vi "INTEGRATION TEST - Legacy Support.vi"(8 "error in (no error)":errorcluster) -> (0 "error out":errorcluster, 2 "Passed":bool)   [LabVIEW 2020, in "test_openg_variant_config_file.lvlib"]
uses:
  test_openg_variant_config_file.lvlib
  <vilib>/Utility/config.llb/NI_LVConfig.lvlib
  source/library/openg_variant_configuration_file.lvlib
  <userlib>/_OpenG.lib/file/file.llb/openg_file.lvlib
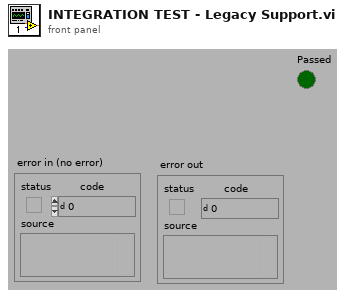
[diagram p1: front panel]
types:
  T1 = typedef "NI_LVConfig.lvlib/Config Data RefNum.ctl" = refnum<k1>
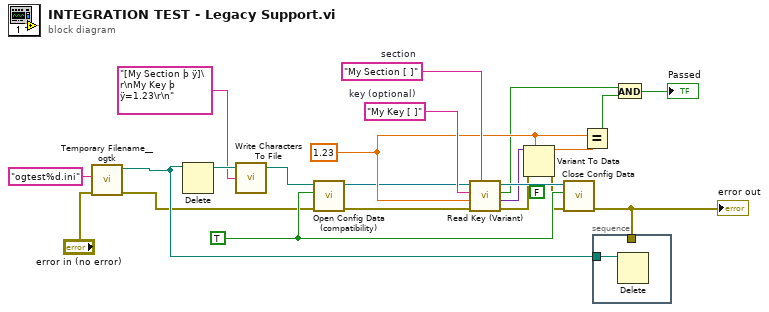
[diagram p0: block diagram]
diagram:
  (unwired) FALSE ("write configuration file? (T)")
  w15 = 1.23 ("Numeric")
  w21 = "My Key [ ]"  # key (optional)
  w22 = "My Section [ ]"  # section
  w19 = TRUE ("create file if necessary? (T)")
  n1 = call <userlib>:"Temporary Filename__ogtk.vi"("error in (no error)"="error in (no error)", "pattern (lvtemp%d.tmp)"="ogtest%d.ini") -> ("error out"=w2:errorcluster, "file in tmp dir"=w3:path)  [unwired: 4 in]
  n2 = Delete(path (use dialog)=w3) -> (deleted path=w9:path)  [unwired: 4 in, 2 out]
  n3 = call <vilib>:"Write Characters To File.vi"("character string"="[My Section þ ÿ]\r\nMy Key þ ÿ=1.23\r\n", "file path (dialog if empty)"=w9) -> ("new file path (Not A Path if cancelled)"=w8:path)  [unwired: 3 in]
  n4 = call <vilib>:"Open Config Data (compatibility).vi"("error in (no error)"=w2, "create file if necessary (T)"=w19, "configuration file path"=w8) -> ("error out"=w5:errorcluster, "refnum"=w6:T1)  [unwired: 6 in, 1 out]
  n5 = call "Read Key (Variant).vi"("section"=w22, "error in (no error)"=w5, "type"=w15, "key (optional)"=w21, "refnum"=w6) -> ("error out"=w16:errorcluster, "key-value"=w18:variant, "found?"=w12:bool, "refnum out"=w20:T1)  [unwired: 3 in]
  n6 = Variant To Data(error in=w16, type=w15, Variant=w18) -> (data=w10:dbl, error out=w17:errorcluster)
  n7 = call <vilib>:"Close Config Data.vi"("error in (no error)"=w17, "write file if changed (T)"=w19, "refnum"=w20) -> ("error out"=w13:errorcluster)  [unwired: 7 in, 1 out]
  "error out" <- w13
  n8 = Equal?(x=w15, y=w10) -> (x = y?=w14:bool)
  n9 = stacked-sequence {
    tunnel: w3 -> [w23]
    tunnel: w13 -> [_]
    frame #0 {
      n10 = Delete(path (use dialog)=w23) -> ()  [unwired: 4 in, 3 out]
    }
  }
  n11 = And(x=w12, y=w14) -> (x .and. y?=→"Passed":bool)
